vi "Make Channels Coincident Low1.vi"(8 "interp. method":i32(ring) items=["nearest", "linear", "spline", "cubic Hermite", "Lagrange"], 9 "Cluster 2":T1={"Colour"=0, "Inst type"=enum."Pitot-static tube", "Inst name"="Manometer voltage", "Symbol"="U", "Code name"="", "Extra Info"="U", "Inst Array"=enum."PWA", "Index"=0, "Voltage Index"=0, "Extra Titles"=[], "Extra Values"=[], "Eng Values"=[], "Time (ms)"=[], "TT / Voltage"=[], "U"=0.0, "u^2"=0.0, "u^3"=0.0, "u^4"=0.0, "Skew_u"=0.0, "Kurt_u"=0.0, "Sd Error in Mean"=0.0, "% u'/U"=0.0, "X"=0.0, "Y"=0.0, "Z"=0.0, "Spectra"={"First Name"="", "Second Name"="", "X axis name"="", "Y axis name"="", "X array"=[], "Y array"=[]}, "Autocorrelation"={"First Name"="", "Second Name"="", "X axis name"="", "Y axis name"="", "X array"=[], "Y array"=[]}, "Timescale integral to 25%"=0.0, "Sd Error in Variance"=0.0, "Calib File"=path "", "Calib Constants"=[], "Histogram"={"First Name"="", "Second Name"="", "X axis name"="", "Y axis name"="", "X array"=[], "Y array"=[]}, "Output Position"=FALSE, "Full Stats"=FALSE} {"Sd Error in Variance" format="%.2f"; "Skew_u" format="%.2f"; "% u'/U" format="%.2f"; "Sd Error in Mean" format="%.2f"; "Kurt_u" format="%.2f"; "u^4" format="%.2f"; "u^3" format="%.2f"; "U" format="%.2f"; "u^2" format="%.2f"}, 11 "Cluster 1":T1={"Colour"=0, "Inst type"=enum."Pitot-static tube", "Inst name"="Manometer voltage", "Symbol"="U", "Code name"="", "Extra Info"="U", "Inst Array"=enum."PWA", "Index"=0, "Voltage Index"=0, "Extra Titles"=[], "Extra Values"=[], "Eng Values"=[], "Time (ms)"=[], "TT / Voltage"=[], "U"=0.0, "u^2"=0.0, "u^3"=0.0, "u^4"=0.0, "Skew_u"=0.0, "Kurt_u"=0.0, "Sd Error in Mean"=0.0, "% u'/U"=0.0, "X"=0.0, "Y"=0.0, "Z"=0.0, "Spectra"={"First Name"="", "Second Name"="", "X axis name"="", "Y axis name"="", "X array"=[], "Y array"=[]}, "Autocorrelation"={"First Name"="", "Second Name"="", "X axis name"="", "Y axis name"="", "X array"=[], "Y array"=[]}, "Timescale integral to 25%"=0.0, "Sd Error in Variance"=0.0, "Calib File"=path "", "Calib Constants"=[], "Histogram"={"First Name"="", "Second Name"="", "X axis name"="", "Y axis name"="", "X array"=[], "Y array"=[]}, "Output Position"=FALSE, "Full Stats"=FALSE} {"Sd Error in Variance" format="%.2f"; "Skew_u" format="%.2f"; "% u'/U" format="%.2f"; "Sd Error in Mean" format="%.2f"; "Kurt_u" format="%.2f"; "u^4" format="%.2f"; "u^3" format="%.2f"; "U" format="%.2f"; "u^2" format="%.2f"}) -> (1 "Coincident Channel 2":T1={"Colour"=0, "Inst type"=enum."Pitot-static tube", "Inst name"="Manometer voltage", "Symbol"="U", "Code name"="", "Extra Info"="U", "Inst Array"=enum."PWA", "Index"=0, "Voltage Index"=0, "Extra Titles"=[], "Extra Values"=[], "Eng Values"=[], "Time (ms)"=[], "TT / Voltage"=[], "U"=0.0, "u^2"=0.0, "u^3"=0.0, "u^4"=0.0, "Skew_u"=0.0, "Kurt_u"=0.0, "Sd Error in Mean"=0.0, "% u'/U"=0.0, "X"=0.0, "Y"=0.0, "Z"=0.0, "Spectra"={"First Name"="", "Second Name"="", "X axis name"="", "Y axis name"="", "X array"=[], "Y array"=[]}, "Autocorrelation"={"First Name"="", "Second Name"="", "X axis name"="", "Y axis name"="", "X array"=[], "Y array"=[]}, "Timescale integral to 25%"=0.0, "Sd Error in Variance"=0.0, "Calib File"=path "", "Calib Constants"=[], "Histogram"={"First Name"="", "Second Name"="", "X axis name"="", "Y axis name"="", "X array"=[], "Y array"=[]}, "Output Position"=FALSE, "Full Stats"=FALSE} {"Sd Error in Variance" format="%.2f"; "Skew_u" format="%.2f"; "% u'/U" format="%.2f"; "Sd Error in Mean" format="%.2f"; "Kurt_u" format="%.2f"; "u^4" format="%.2f"; "u^3" format="%.2f"; "U" format="%.2f"; "u^2" format="%.2f"}, 3 "Coincident Channel 1":T1={"Colour"=0, "Inst type"=enum."Pitot-static tube", "Inst name"="Manometer voltage", "Symbol"="U", "Code name"="", "Extra Info"="U", "Inst Array"=enum."PWA", "Index"=0, "Voltage Index"=0, "Extra Titles"=[], "Extra Values"=[], "Eng Values"=[], "Time (ms)"=[], "TT / Voltage"=[], "U"=0.0, "u^2"=0.0, "u^3"=0.0, "u^4"=0.0, "Skew_u"=0.0, "Kurt_u"=0.0, "Sd Error in Mean"=0.0, "% u'/U"=0.0, "X"=0.0, "Y"=0.0, "Z"=0.0, "Spectra"={"First Name"="", "Second Name"="", "X axis name"="", "Y axis name"="", "X array"=[], "Y array"=[]}, "Autocorrelation"={"First Name"="", "Second Name"="", "X axis name"="", "Y axis name"="", "X array"=[], "Y array"=[]}, "Timescale integral to 25%"=0.0, "Sd Error in Variance"=0.0, "Calib File"=path "", "Calib Constants"=[], "Histogram"={"First Name"="", "Second Name"="", "X axis name"="", "Y axis name"="", "X array"=[], "Y array"=[]}, "Output Position"=FALSE, "Full Stats"=FALSE} {"Sd Error in Variance" format="%.2f"; "Skew_u" format="%.2f"; "% u'/U" format="%.2f"; "Sd Error in Mean" format="%.2f"; "Kurt_u" format="%.2f"; "u^4" format="%.2f"; "u^3" format="%.2f"; "U" format="%.2f"; "u^2" format="%.2f"})   [LabVIEW 2011]
uses:
  Controls/Analysis_info_cluster.ctl
  Controls/Inst_type.ctl
  Controls/Instrument_Array.ctl
  Controls/XY_Plot_Cluster.ctl
  <vilib>/gmath/NI_Gmath.lvlib
panel:
  in  "Show Plots":bool
  out "Start Time":dbl
  out "End Time":dbl
  out "U1 and U2 Raw":cluster{"yi":dbl[], "yi":dbl[]}[](graph)
  out "U1 and U2 made coincident":cluster{"yi":dbl[], "yi":dbl[]}[](graph)
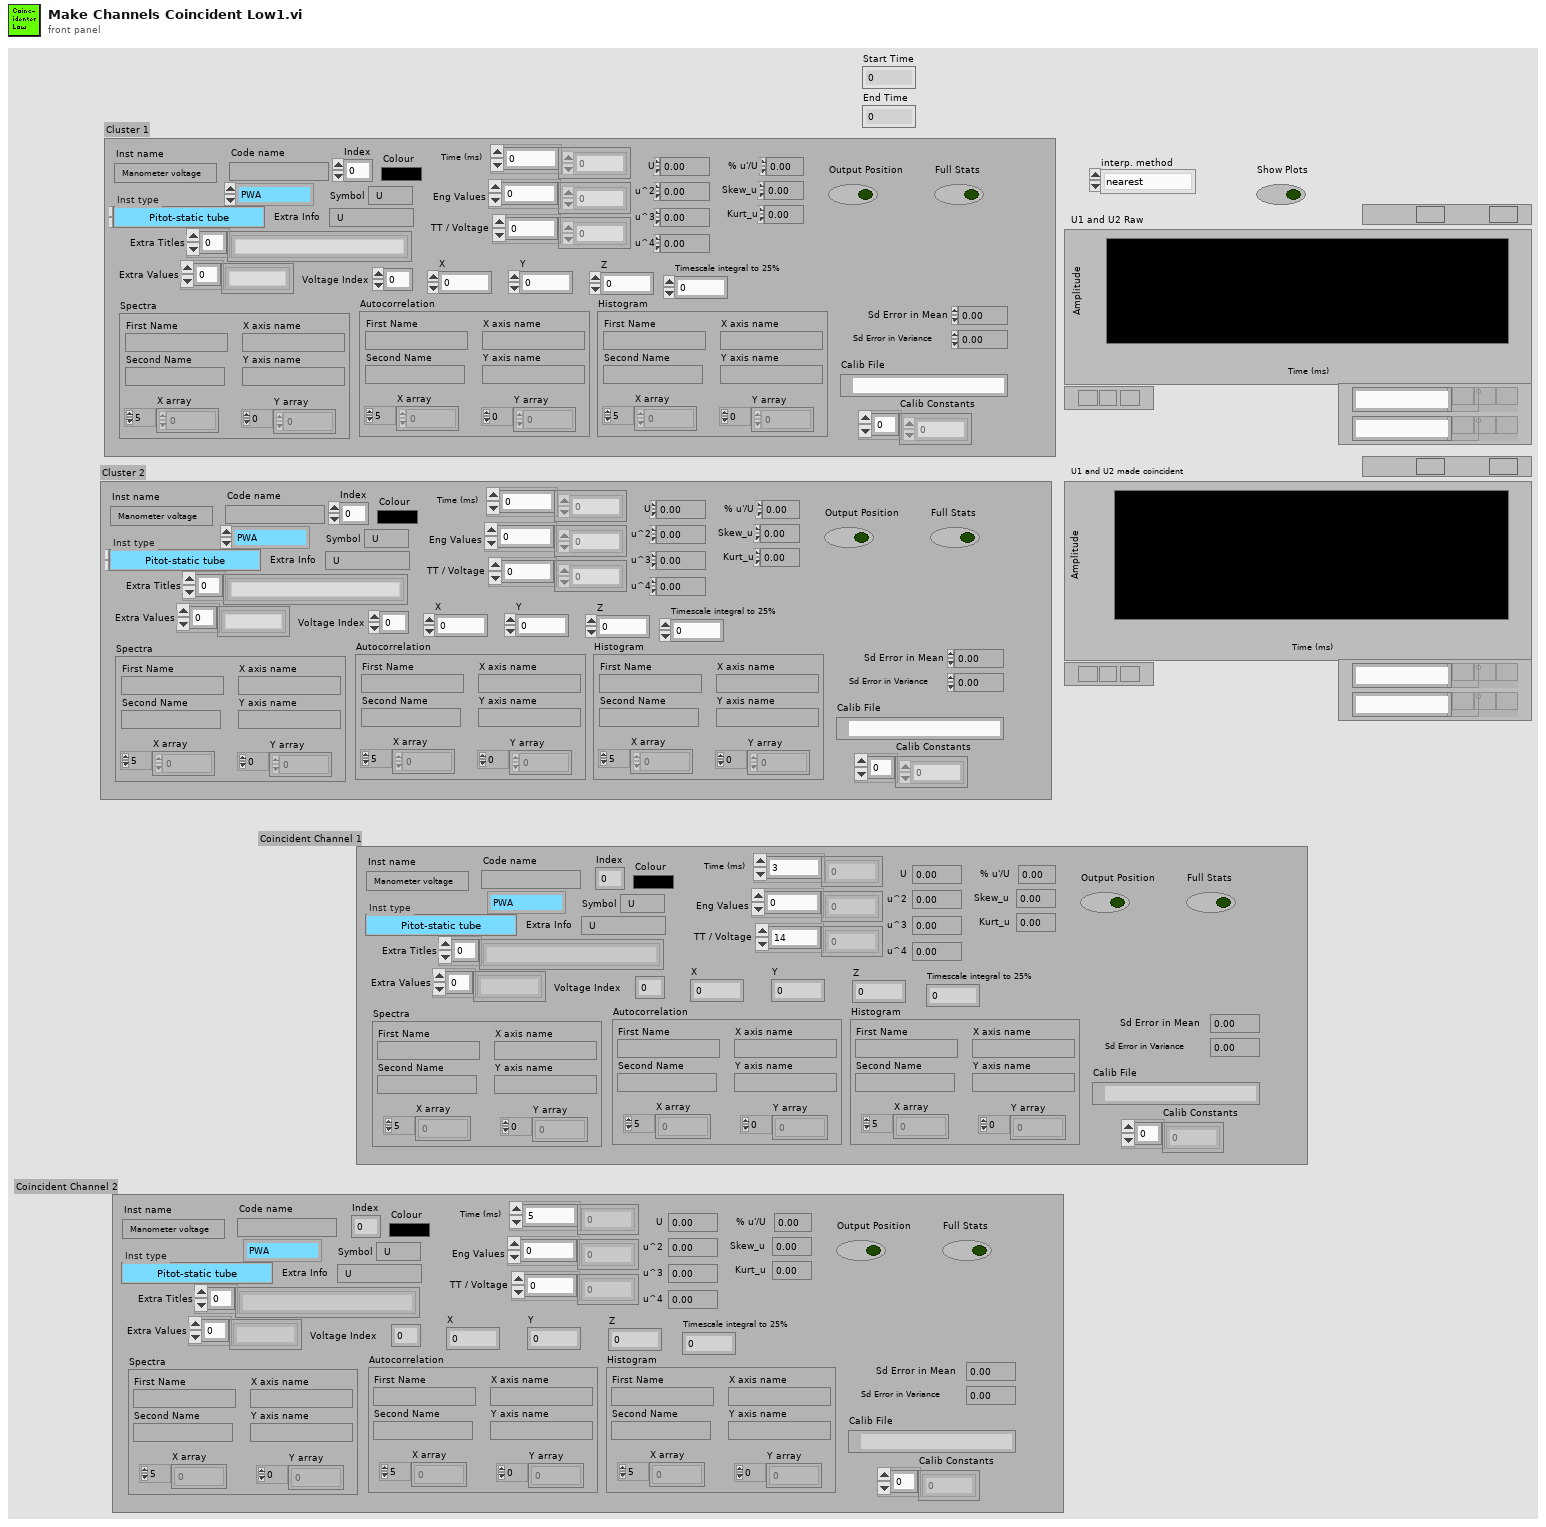
[diagram p1: front panel]
types:
  T1 = typedef "Analysis_info_cluster.ctl" = cluster{"Colour":u32, "Inst type":T2, "Inst name":string, "Symbol":string, "Code name":string, "Extra Info":string, "Inst Array":T3, "Index":i32, "Voltage Index":i32, "Extra Titles":string[], "Extra Values":string[], "Eng Values":dbl[], "Time (ms)":dbl[], "TT / Voltage":dbl[], "U":dbl, "u^2":dbl, "u^3":dbl, "u^4":dbl, "Skew_u":dbl, "Kurt_u":dbl, "Sd Error in Mean":dbl, "% u'/U":dbl, "X":dbl, "Y":dbl, "Z":dbl, "Spectra":T4, "Autocorrelation":T4, "Timescale integral to 25%":dbl, "Sd Error in Variance":dbl, "Calib File":path, "Calib Constants":dbl[], "Histogram":T4, "Output Position":bool, "Full Stats":bool}
  T2 = typedef "Inst_type.ctl" = enum16{"Propeller anemometer", "Raw voltage", "Pressure Transducer", "Pitot-static tube", "Preston tube", "Hot wire", "Cross wire 1", "Cross wire 2", "Generic Linear", "Generic Polynomial", "Generic BackPoly", "Fast FID", "Thermocouple", "Cold wire", "Pulsed Wire", "LDA Vel", "LDA Tran time", "LDA Arr time"}
  T3 = typedef "Instrument_Array.ctl" = enum16{"PWA", "LDA", "Analogue"}
  T4 = typedef "XY_Plot_Cluster.ctl" = cluster{"First Name":string, "Second Name":string, "X axis name":string, "Y axis name":string, "X array":dbl[], "Y array":dbl[]}
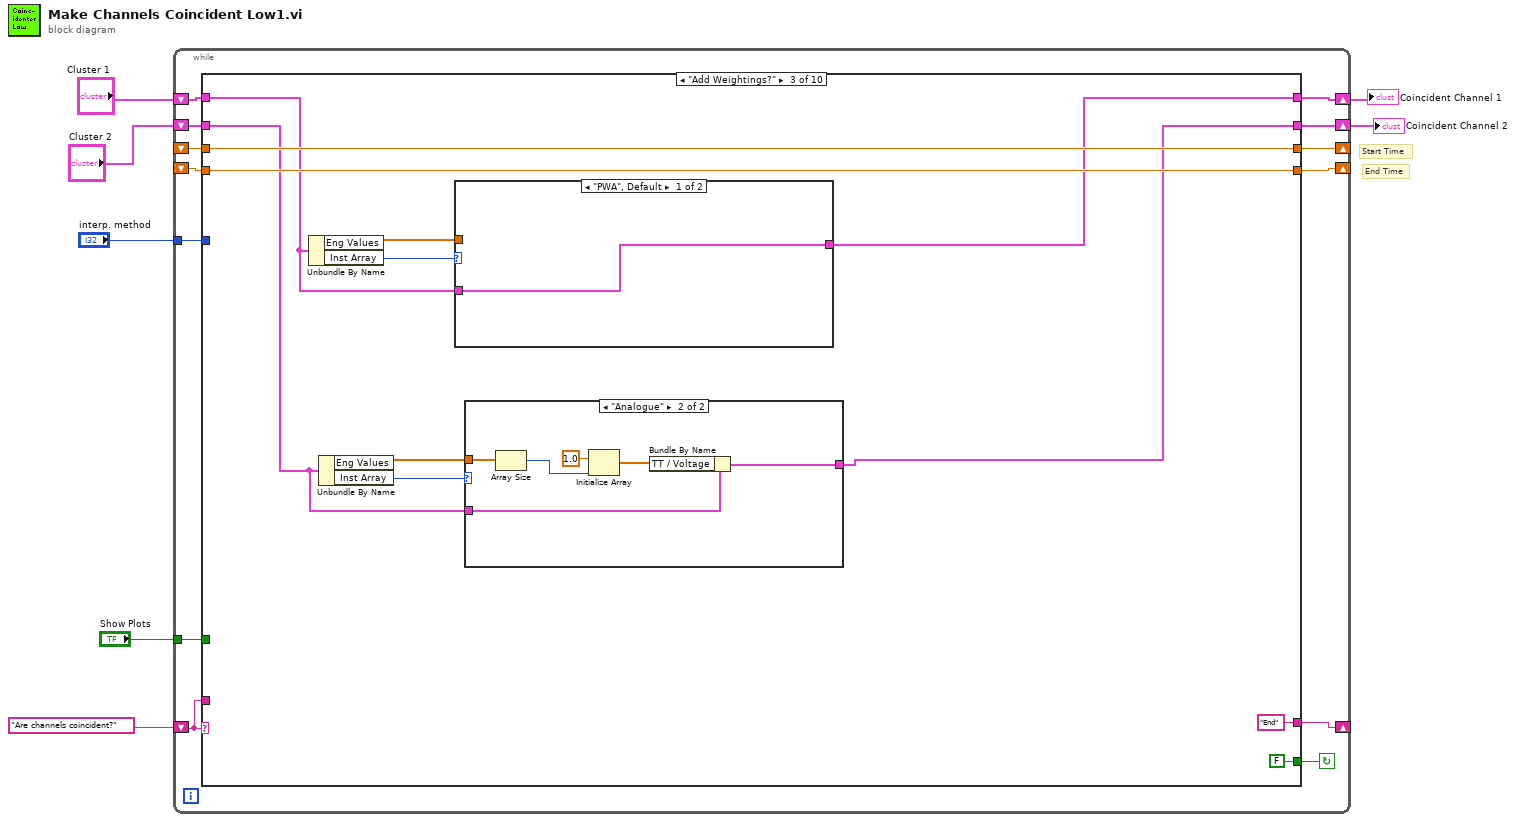
[diagram p0: block diagram]
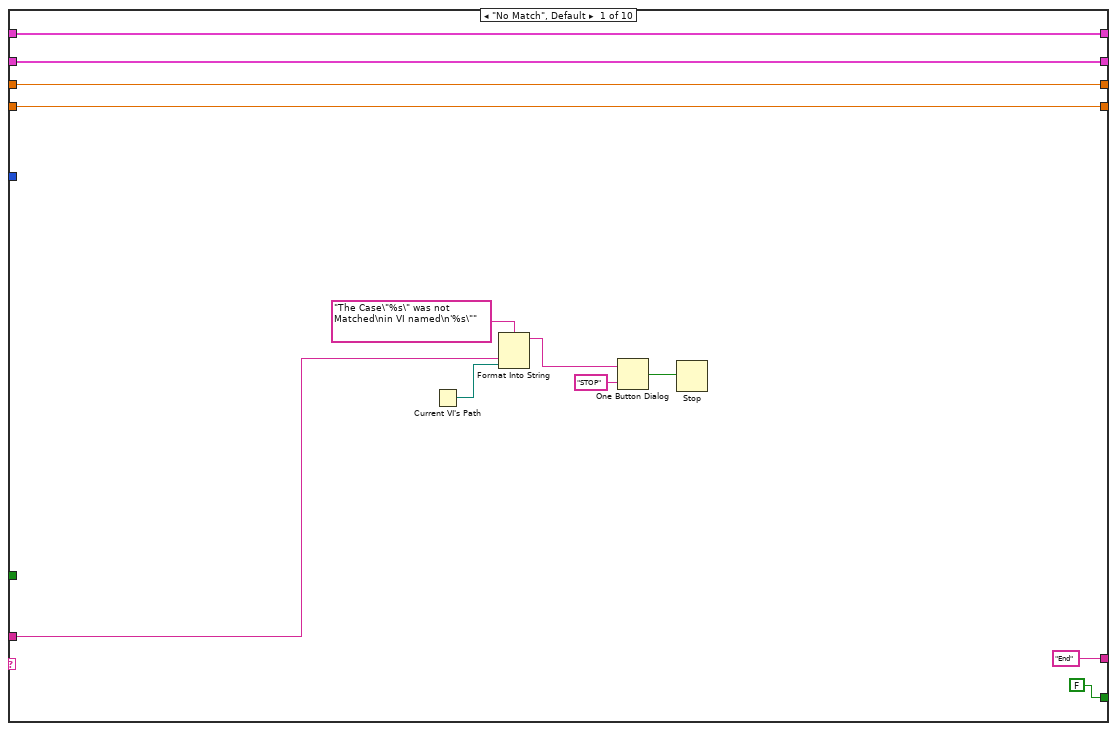
[diagram p2: hidden frame]
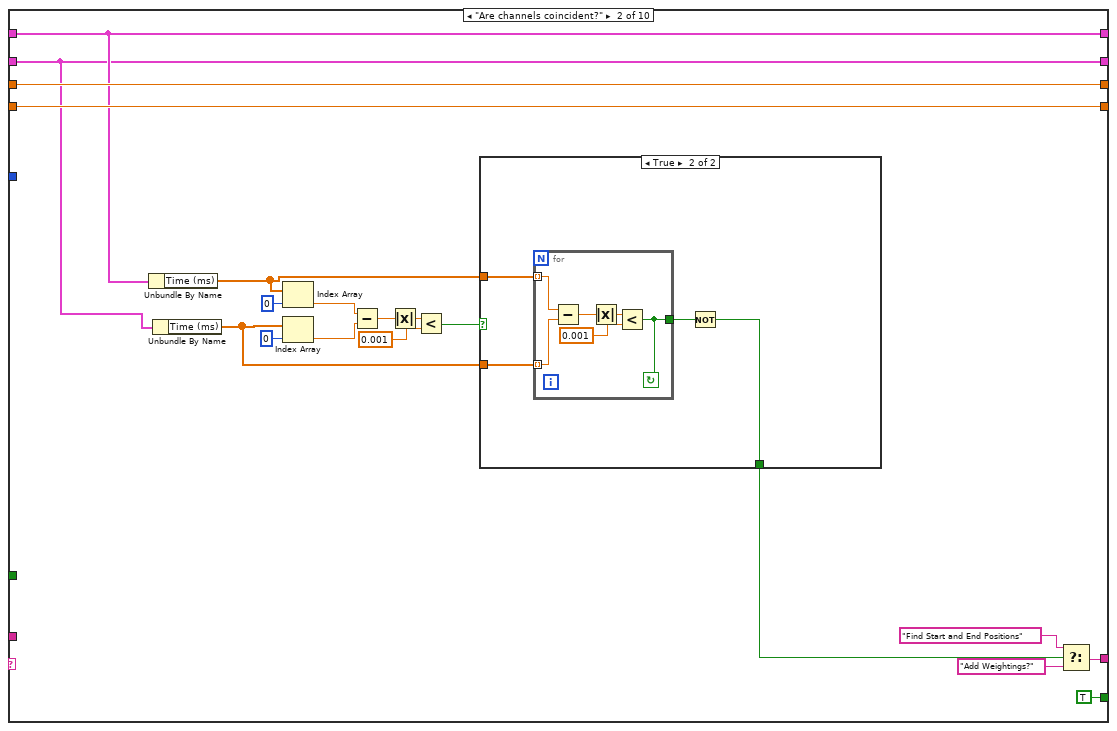
[diagram p3: hidden frame]
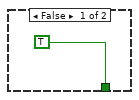
[diagram p4: hidden frame]
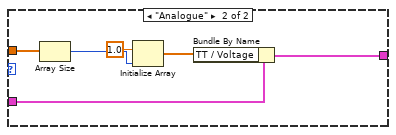
[diagram p6: hidden frame]
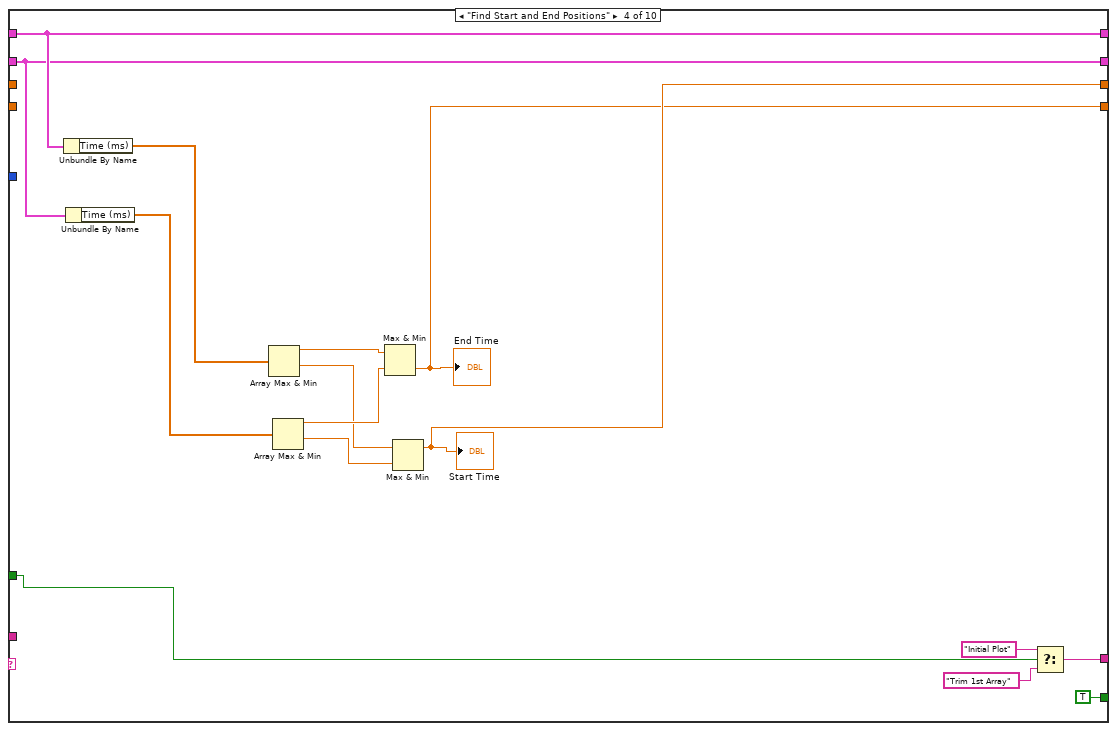
[diagram p7: hidden frame]
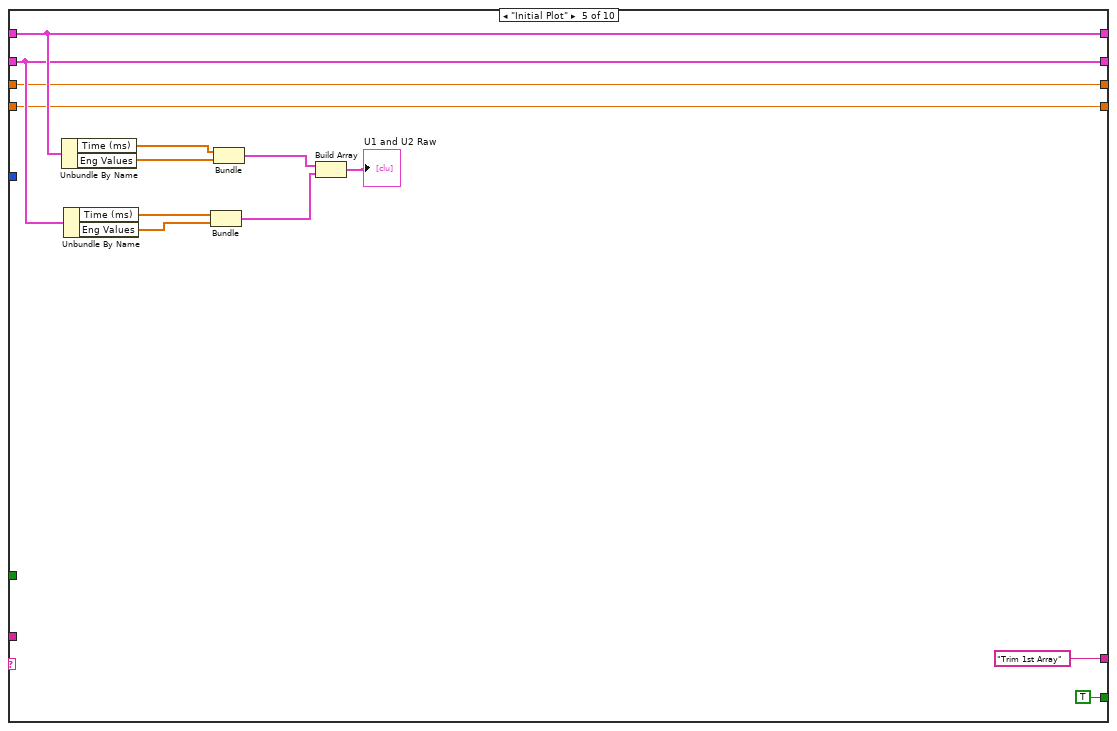
[diagram p8: hidden frame]
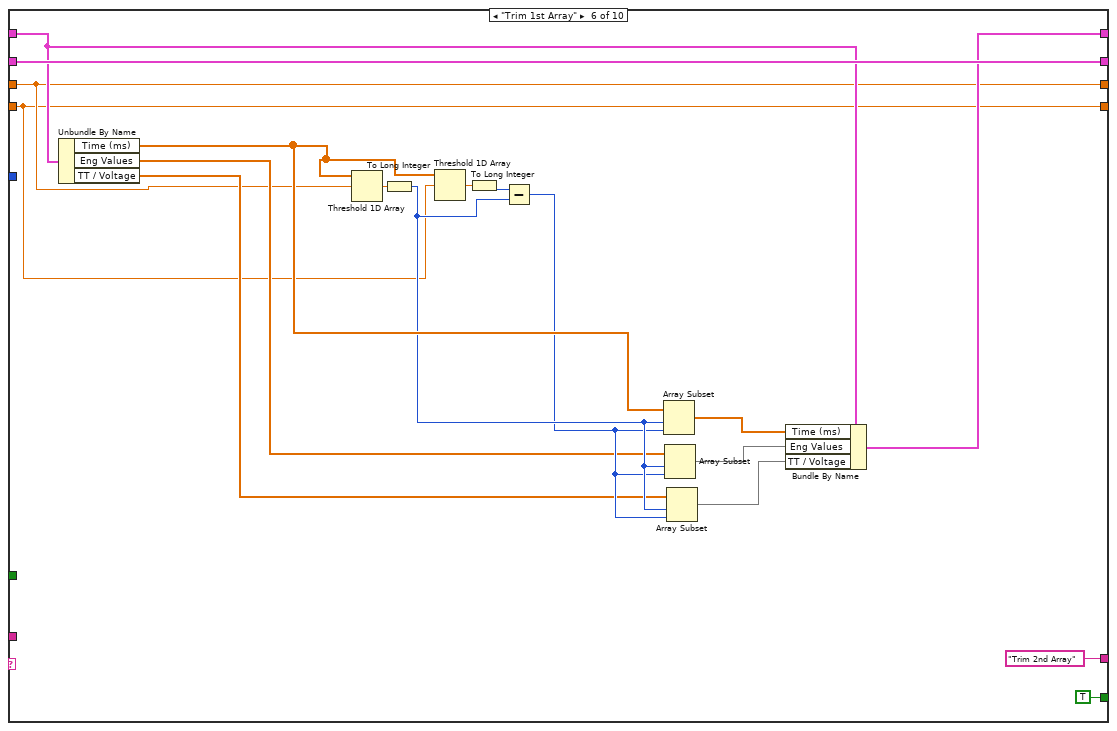
[diagram p9: hidden frame]
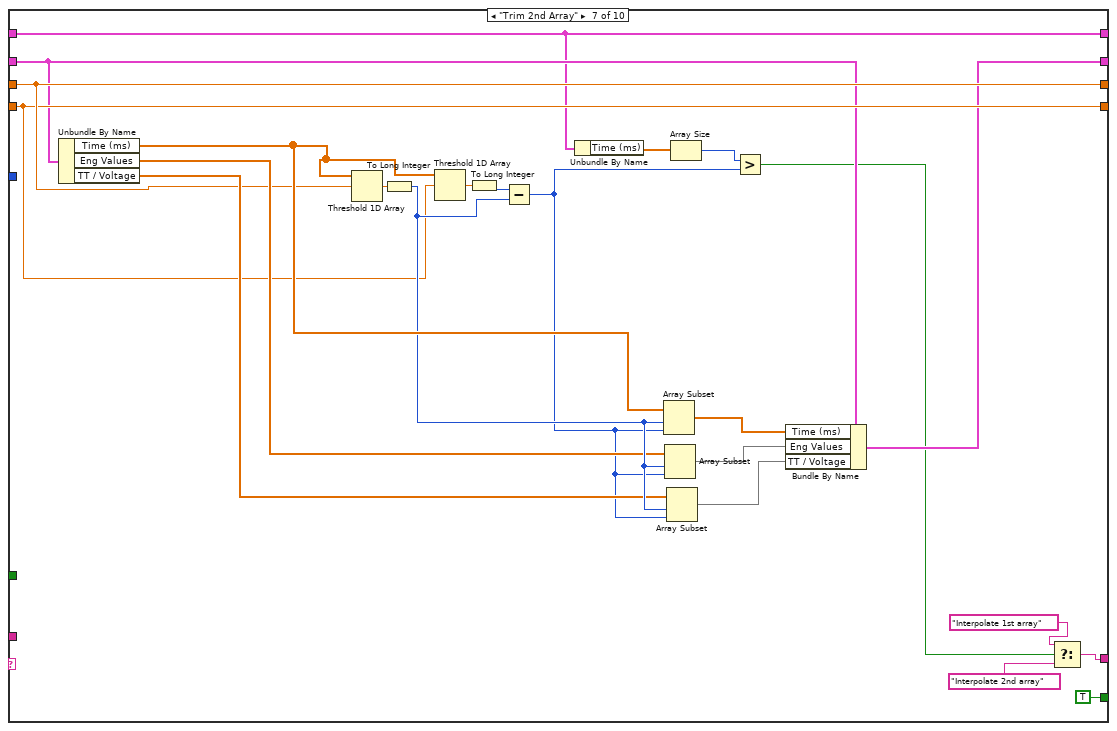
[diagram p10: hidden frame]
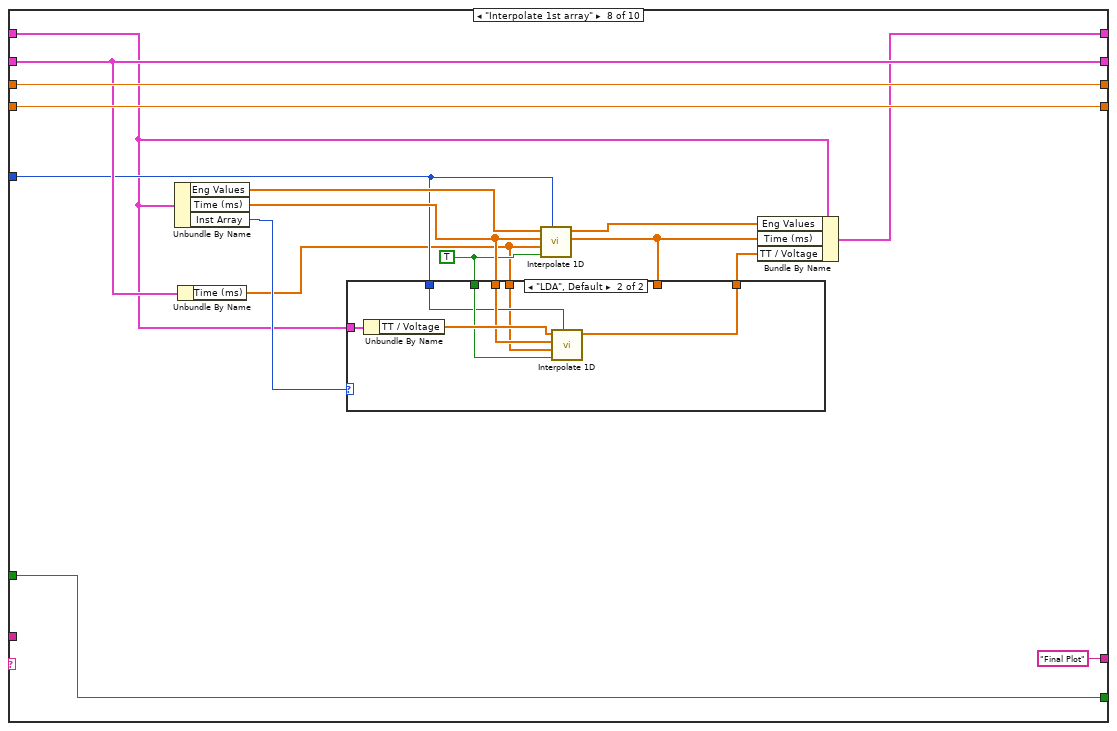
[diagram p11: hidden frame]
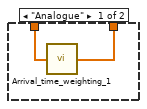
[diagram p12: hidden frame]
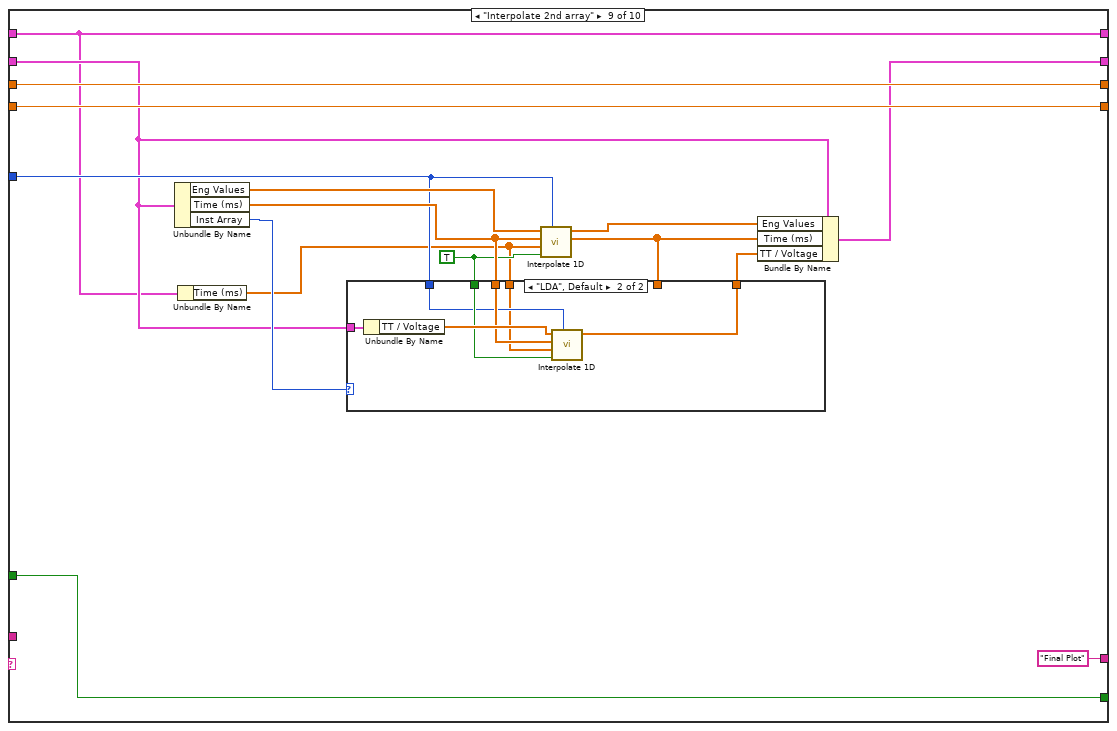
[diagram p13: hidden frame]
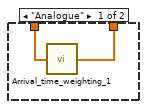
[diagram p14: hidden frame]
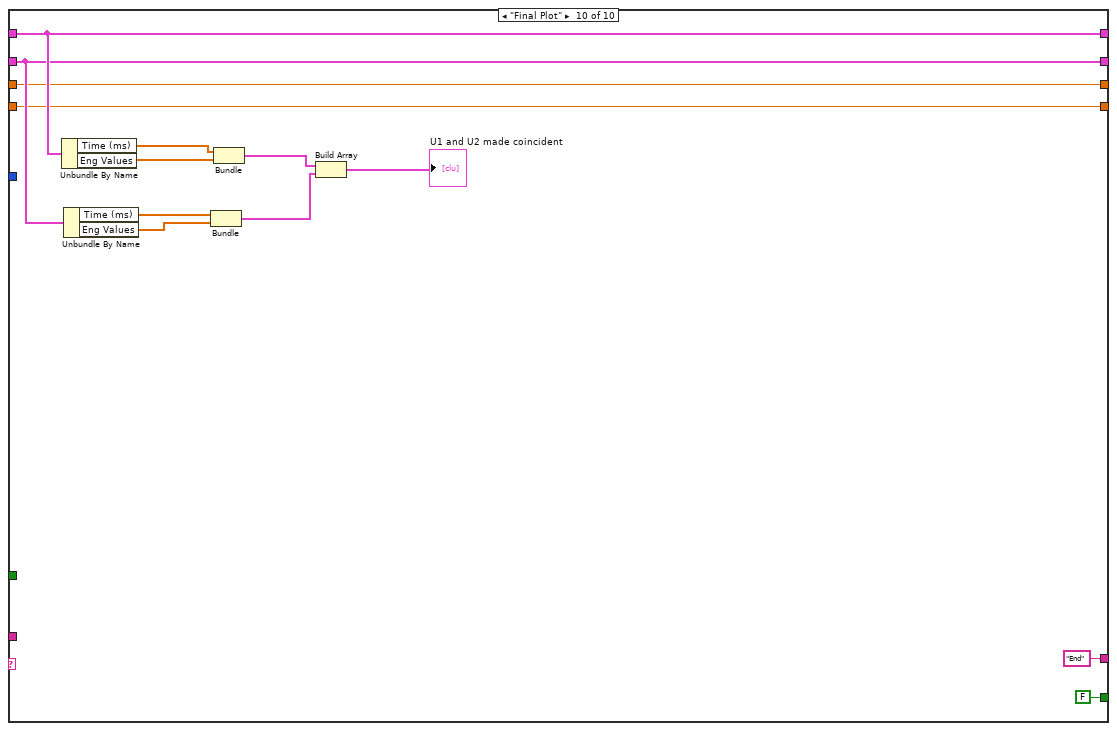
[diagram p15: hidden frame]
diagram:
  # "End Time"
  # "Start Time"
  n1 = while {
    shift-right: [w15] -> w2
    shift-left: "Cluster 1" -> [w17]
    shift-right: [w14] -> w3
    shift-left: "Cluster 2" -> [w16]
    shift-right: [w18] -> _
    shift-left: "Are channels coincident?" -> [w20]
    shift-right: [w12] -> _
    shift-left: _ -> [w13]
    shift-right: [w11] -> _
    shift-left: _ -> [w10]
    tunnel: "interp. method" -> [w9]
    tunnel: "Show Plots" -> [w8]
    stop <- w19 continue-if-true
    n2 = case shown="\"Add Weightings?\"" w20 {
      tunnel: w20 -> [w27 _ _ _ _ _ _ _ _ _]
      tunnel: [FALSE TRUE ("Show Plots") FALSE ("Show Plots") TRUE TRUE TRUE TRUE w159 w187 FALSE] -> w19
      tunnel: ["End" w33 "End" ("t") w90 "Trim 1st Array" "Trim 2nd Array" w135 "Final Plot" "Final Plot" "End" ("t")] -> w18
      tunnel: w17 -> [w24 w42 w69 w102 w115 w130 w143 w162 w183 w219]
      tunnel: w16 -> [w23 w41 w64 w101 w114 w133 w144 w171 w185 w218]
      tunnel: [w24 w42 w67 w102 w115 w120 w143 w166 w183 w219] -> w15
      tunnel: [w23 w41 w63 w101 w114 w133 w145 w171 w184 w218] -> w14
      tunnel: w13 -> [w22 w51 w74 _ w106 w119 w147 w173 w198 w211]
      tunnel: [w22 w51 w74 w94 w106 w119 w147 w173 w198 w211] -> w12
      tunnel: [w21 w50 w73 w93 w105 w118 w146 w172 w197 w210] -> w11
      tunnel: w10 -> [w21 w50 w73 _ w105 w118 w146 w172 w197 w210]
      tunnel: w9 -> [_ _ _ _ _ _ _ w164 w191 _]
      tunnel: w8 -> [_ _ _ w92 _ _ _ w159 w187 _]
      frame "No Match", Default {
        n3 = Current VI's Path() -> (path=w32:path)
        n4 = Format Into String(format string="The Case\"%s\" was not Matched\nin VI named\n'%s\"" ("Format String"), w27, w32) -> (resulting string=w29:string)  [unwired: 2 in, 1 out]
        n5 = One Button Dialog(message=w29, button name ("OK")="STOP") -> (true=w31:bool)
        n6 = Stop(stop? (T)=w31) -> ()
      }
      frame "Are channels coincident?" {
        n7 = Unbundle By Name(w42) -> ("Time (ms)"=w39:dbl[])
        n8 = Unbundle By Name(w41) -> ("Time (ms)"=w38:dbl[])
        n9 = Index Array(array=w39, index=0) -> (element=w45:dbl)
        n10 = Index Array(array=w38, index=0) -> (element=w46:dbl)
        n11 = Subtract(x=w45, y=w46) -> (x-y=w47:dbl)
        n12 = Absolute Value(x=w47) -> (abs(x)=w48:dbl)
        n13 = Less?(x=w48, y=0.001) -> (x < y?=w40:bool)
        n14 = case shown="True" w40 {
          tunnel: w39 -> [_ w56]
          tunnel: w38 -> [_ w55]
          tunnel: [TRUE w53] -> w36
          frame False {
          }
          frame True {
            n15 = for {
              tunnel: w56 -> [w59] mode=indexing
              tunnel: w55 -> [w58] mode=indexing
              tunnel: [w57] -> w54
              stop <- w57 continue-if-true
              n16 = Subtract(x=w59, y=w58) -> (x-y=w62:dbl)
              n17 = Absolute Value(x=w62) -> (abs(x)=w61:dbl)
              n18 = Less?(x=w61, y=0.001) -> (x < y?=w57:bool)
            }
            n19 = Not(x=w54) -> (.not. x?=w53:bool)
          }
        }
        n20 = Select(t="Find Start and End Positions", s=w36, f="Add Weightings?") -> (s? t:f=w33:string)
      }
      frame "Add Weightings?" {
        n21 = Unbundle By Name(w69) -> ("Eng Values"=w68:dbl[], "Inst Array"=w70:T3)
        n22 = Unbundle By Name(w64) -> ("Eng Values"=w66:dbl[], "Inst Array"=w65:T3)
        n23 = case shown="\"PWA\", Default" w70 {
          tunnel: w69 -> [w82 w88]
          tunnel: w68 -> [_ w87]
          tunnel: [w82 w83] -> w67
          frame "PWA", Default {
          }
          frame "Analogue" {
            n24 = Array Size(array=w87) -> (size(s)=w86:i32)
            n25 = Initialize Array(1.0 ("element"), w86) -> (w84:dbl[])
            n26 = Bundle By Name(cluster=w88, "TT / Voltage"=w84) -> (w83:T1)
          }
        }
        n27 = case shown="\"Analogue\"" w65 {
          tunnel: w64 -> [w75 w81]
          tunnel: w66 -> [_ w80]
          tunnel: [w75 w76] -> w63
          frame "PWA", Default {
          }
          frame "Analogue" {
            n28 = Array Size(array=w80) -> (size(s)=w79:i32)
            n29 = Initialize Array(1.0 ("element"), w79) -> (w77:dbl[])
            n30 = Bundle By Name(cluster=w81, "TT / Voltage"=w77) -> (w76:T1)
          }
        }
      }
      frame "Find Start and End Positions" {
        n31 = Unbundle By Name(w102) -> ("Time (ms)"=w95:dbl[])
        n32 = Unbundle By Name(w101) -> ("Time (ms)"=w100:dbl[])
        n33 = Array Max & Min(array=w95) -> (max value=w99:dbl, min value=w97:dbl)  [unwired: 2 out]
        n34 = Array Max & Min(array=w100) -> (max value=w98:dbl, min value=w96:dbl)  [unwired: 2 out]
        n35 = Max & Min(x=w99, y=w98) -> (min(x,y)=w93:dbl)  [unwired: 1 out]
        "End Time" <- w93
        n36 = Max & Min(x=w97, y=w96) -> (max(x,y)=w94:dbl)  [unwired: 1 out]
        "Start Time" <- w94
        n37 = Select(t="Initial Plot", s=w92, f="Trim 1st Array") -> (s? t:f=w90:string)
      }
      frame "Initial Plot" {
        n38 = Unbundle By Name(w115) -> ("Time (ms)"=w107:dbl[], "Eng Values"=w111:dbl[])
        n39 = Unbundle By Name(w114) -> ("Time (ms)"=w108:dbl[], "Eng Values"=w110:dbl[])
        n40 = Bundle("Time (ms)"=w108, "Eng Values"=w110) -> (w109:cluster{"Time (ms)":dbl[], "Eng Values":dbl[]})  [unwired: 1 in]
        n41 = Bundle("Time (ms)"=w107, "Eng Values"=w111) -> (w112:cluster{"Time (ms)":dbl[], "Eng Values":dbl[]})  [unwired: 1 in]
        n42 = Build Array(w112, w109) -> (→"U1 and U2 Raw":cluster{"Time (ms)":dbl[], "Eng Values":dbl[]}[])
      }
      frame "Trim 1st Array" {
        n43 = Unbundle By Name(w130) -> ("Time (ms)"=w129:dbl[], "Eng Values"=w125:dbl[], "TT / Voltage"=w124:dbl[])
        n44 = Threshold 1D Array(2:w119, 3:w129) -> (0:w131:dbl)  [unwired: 1 in]
        n45 = To Long Integer(number=w131) -> (32bit integer=w127:i32)
        n46 = Threshold 1D Array(2:w118, 3:w129) -> (0:w132:dbl)  [unwired: 1 in]
        n47 = To Long Integer(number=w132) -> (32bit integer=w128:i32)
        n48 = Subtract(x=w128, y=w127) -> (x-y=w126:i32)
        n49 = Array Subset(array=w129, index=w127, length=w126) -> (w123:dbl[])
        n50 = Array Subset(array=w125, index=w127, length=w126) -> (w122:dbl[])
        n51 = Array Subset(array=w124, index=w127, length=w126) -> (w121:dbl[])
        n52 = Bundle By Name(cluster=w130, "Time (ms)"=w123, "Eng Values"=w122, "TT / Voltage"=w121) -> (w120:T1)
      }
      frame "Trim 2nd Array" {
        n53 = Unbundle By Name(w144) -> ("Time (ms)"=w154:dbl[], "Eng Values"=w151:dbl[], "TT / Voltage"=w150:dbl[])
        n54 = Threshold 1D Array(2:w147, 3:w154) -> (0:w155:dbl)  [unwired: 1 in]
        n55 = To Long Integer(number=w155) -> (32bit integer=w152:i32)
        n56 = Threshold 1D Array(2:w146, 3:w154) -> (0:w156:dbl)  [unwired: 1 in]
        n57 = To Long Integer(number=w156) -> (32bit integer=w153:i32)
        n58 = Subtract(x=w153, y=w152) -> (x-y=w139:i32)
        n59 = Unbundle By Name(w143) -> ("Time (ms)"=w142:dbl[])
        n60 = Array Subset(array=w154, index=w152, length=w139) -> (w141:dbl[])
        n61 = Array Subset(array=w151, index=w152, length=w139) -> (w149:dbl[])
        n62 = Array Subset(array=w150, index=w152, length=w139) -> (w148:dbl[])
        n63 = Array Size(array=w142) -> (size(s)=w140:i32)
        n64 = Greater?(x=w140, y=w139) -> (0:w138:bool)
        n65 = Bundle By Name(cluster=w144, "Time (ms)"=w141, "Eng Values"=w149, "TT / Voltage"=w148) -> (w145:T1)
        n66 = Select(t="Interpolate 1st array", s=w138, f="Interpolate 2nd array") -> (s? t:f=w135:string)
      }
      frame "Interpolate 1st array" {
        w165 = TRUE ("X is monotonic")
        n67 = Unbundle By Name(w162) -> ("Eng Values"=w170:dbl[], "Time (ms)"=w167:dbl[], "Inst Array"=w168:T3)
        n68 = Unbundle By Name(w171) -> ("Time (ms)"=w163:dbl[])
        n69 = call <vilib>:"Interpolate 1D.vi"("method"=w164, "X is monotonic"=w165, "xi"=w163, "X"=w167, "Y"=w170) -> ("xi used"=w160:dbl[], "yi"=w169:dbl[])  [unwired: 1 in, 4 out]
        n70 = case shown="\"LDA\", Default" w168 {
          tunnel: w162 -> [_ w180]
          tunnel: w167 -> [_ w181]
          tunnel: w165 -> [_ w179]
          tunnel: w164 -> [_ w178]
          tunnel: w163 -> [_ w177]
          tunnel: [w174 w176] -> w161
          tunnel: w160 -> [w175 _]
          frame "Analogue" {
            n71 = call "Arrival_time_weighting_1.vi"("Arrival times"=w175) -> ("Weighting"=w174:dbl[])
          }
          frame "LDA", Default {
            n72 = Unbundle By Name(w180) -> ("TT / Voltage"=w182:dbl[])
            n73 = call <vilib>:"Interpolate 1D.vi"("method"=w178, "X is monotonic"=w179, "xi"=w177, "X"=w181, "Y"=w182) -> ("yi"=w176:dbl[])  [unwired: 1 in, 5 out]
          }
        }
        n74 = Bundle By Name(cluster=w162, "Eng Values"=w169, "Time (ms)"=w160, "TT / Voltage"=w161) -> (w166:T1)
      }
      frame "Interpolate 2nd array" {
        w192 = TRUE ("X is monotonic")
        n75 = Unbundle By Name(w185) -> ("Eng Values"=w196:dbl[], "Time (ms)"=w193:dbl[], "Inst Array"=w194:T3)
        n76 = Unbundle By Name(w183) -> ("Time (ms)"=w190:dbl[])
        n77 = call <vilib>:"Interpolate 1D.vi"("method"=w191, "X is monotonic"=w192, "xi"=w190, "X"=w193, "Y"=w196) -> ("xi used"=w188:dbl[], "yi"=w195:dbl[])  [unwired: 1 in, 4 out]
        n78 = case shown="\"LDA\", Default" w194 {
          tunnel: w185 -> [_ w205]
          tunnel: w193 -> [_ w206]
          tunnel: w192 -> [_ w204]
          tunnel: w191 -> [_ w203]
          tunnel: w190 -> [_ w202]
          tunnel: [w199 w201] -> w189
          tunnel: w188 -> [w200 _]
          frame "Analogue" {
            n79 = call "Arrival_time_weighting_1.vi"("Arrival times"=w200) -> ("Weighting"=w199:dbl[])
          }
          frame "LDA", Default {
            n80 = Unbundle By Name(w205) -> ("TT / Voltage"=w207:dbl[])
            n81 = call <vilib>:"Interpolate 1D.vi"("method"=w203, "X is monotonic"=w204, "xi"=w202, "X"=w206, "Y"=w207) -> ("yi"=w201:dbl[])  [unwired: 1 in, 5 out]
          }
        }
        n82 = Bundle By Name(cluster=w185, "Eng Values"=w195, "Time (ms)"=w188, "TT / Voltage"=w189) -> (w184:T1)
      }
      frame "Final Plot" {
        n83 = Unbundle By Name(w219) -> ("Time (ms)"=w212:dbl[], "Eng Values"=w216:dbl[])
        n84 = Unbundle By Name(w218) -> ("Time (ms)"=w213:dbl[], "Eng Values"=w215:dbl[])
        n85 = Bundle("Time (ms)"=w213, "Eng Values"=w215) -> (w214:cluster{"Time (ms)":dbl[], "Eng Values":dbl[]})  [unwired: 1 in]
        n86 = Bundle("Time (ms)"=w212, "Eng Values"=w216) -> (w217:cluster{"Time (ms)":dbl[], "Eng Values":dbl[]})  [unwired: 1 in]
        n87 = Build Array(w217, w214) -> (→"U1 and U2 made coincident":cluster{"Time (ms)":dbl[], "Eng Values":dbl[]}[])
      }
    }
  }
  "Coincident Channel 1" <- w2
  "Coincident Channel 2" <- w3
